vi "ConvertCountsToSI.vi"(7 "Scale Factor":dbl, 8 "Count Array 3":i16[](array[numeric]), 9 "Count Array 2":i16[](array[numeric]), 10 "Count Array 1":i16[](array[numeric]), 11 "Count Array 0":i16[](array[numeric])) -> (0 "SI Array 3":dbl[](array[numeric]), 1 "SI Array 2":dbl[](array[numeric]), 2 "SI Array 1":dbl[](array[numeric]), 3 "SI Array 0":dbl[](array[numeric]))   [LabVIEW 2014]
doc: "Convert Counts to SI units (V) by mulitplying by scale factors."
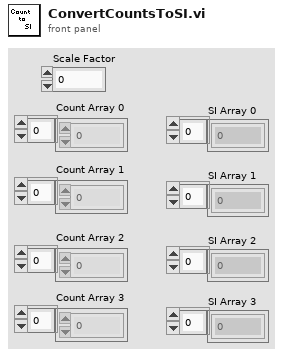
[diagram p1: front panel]
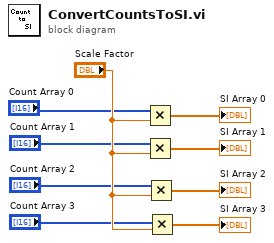
[diagram p0: block diagram]
diagram:
  n1 = Multiply(x="Count Array 0", y="Scale Factor") -> (x*y=→"SI Array 0":dbl[])
  n2 = Multiply(x="Count Array 1", y="Scale Factor") -> (x*y=→"SI Array 1":dbl[])
  n3 = Multiply(x="Count Array 2", y="Scale Factor") -> (x*y=→"SI Array 2":dbl[])
  n4 = Multiply(x="Count Array 3", y="Scale Factor") -> (x*y=→"SI Array 3":dbl[])
